vi "FTW-System-CurrentProcessResourceUsage.vi"(11 "error in":errorcluster) -> (2 "Hard Page Faults":u64 format="%d kilobytes", 3 "LabVIEW Dataspace Size":u64 format="%d kilobytes", 4 "Processor Time (Userspace)":dbl format="%.3fsec", 6 "Processor Time (System)":dbl format="%.3fsec", 8 "Current High-Resolution Timer":dbl format="%.6fsec", 10 "Peak Working Set Size":u64 format="%d kilobytes", 14 "System Uptime":dbl format="%.3fmsec\n%<%D:%H:%M:%S%3u>t", 15 "error out":errorcluster)   [LabVIEW 2015]
panel:
  # "Inputs"
  # "Outputs"
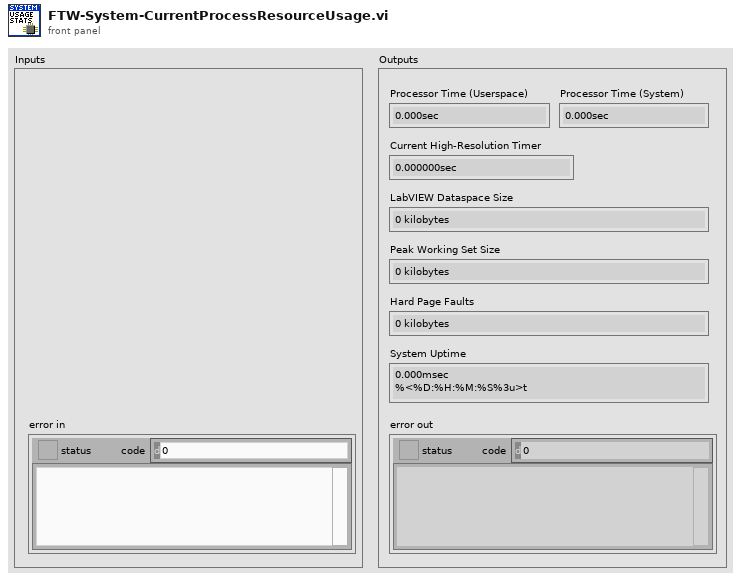
[diagram p1: front panel]
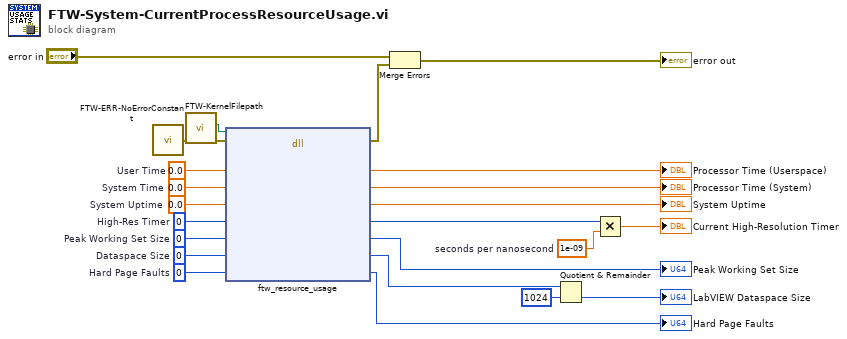
[diagram p0: block diagram]
diagram:
  w2 = 0.0  # System Uptime
  w4 = 1e-09  # seconds per nanosecond
  w6 = u64 0  # High-Res Timer
  w15 = u64 0  # Dataspace Size
  w22 = u64 0  # Hard Page Faults
  w21 = u64 0  # Peak Working Set Size
  w20 = 0.0  # System Time
  w19 = 0.0  # User Time
  n1 = call "FTW-ERR-NoErrorConstant.vi"() -> ("no error"=w16:errorcluster)
  n2 = call "FTW-KernelFilepath.vi"("error in"=w16) -> ("error out"=w17:errorcluster, "Library Filepath"=w18:path)  [unwired: 8 in, 1 out]
  n3 = dll-call lib="?" fn="ftw_resource_usage"(path in=w18, error in=w17, "User Time"=w19, "System Time"=w20, "System Uptime"=w2, "High-Res Timer"=w6, "Peak Working Set Size"=w21, "Dataspace Size"=w15, "Hard Page Faults"=w22) -> (error out=w14:errorcluster, "User Time"=→"Processor Time (Userspace)":dbl, "System Time"=→"Processor Time (System)":dbl, "System Uptime"=→"System Uptime":dbl, "High-Res Timer"=w5:u64, "Peak Working Set Size"=→"Peak Working Set Size":u64, "Dataspace Size"=w9:u64, "Hard Page Faults"=→"Hard Page Faults":u64)  [unwired: 2 in, 1 out]
  n4 = Merge Errors("error in", w14) -> (→"error out":errorcluster)
  n5 = Quotient & Remainder(x=w9, y=u64 1024) -> (floor(x/y)=→"LabVIEW Dataspace Size":u64)  [unwired: 1 out]
  n6 = Multiply(x=w5, y=w4) -> (x*y=→"Current High-Resolution Timer":dbl)
